vi "Write Base Actor DVR.vi"(10 "Base Actor DVR":refnum<data-value>, 11 "TEMPLATE Actor in":refnum<class "TEMPLATE Actor.lvclass">) -> (3 "TEMPLATE Actor out":refnum<class "TEMPLATE Actor.lvclass">)   [LabVIEW 2020, in "_Template.lvlib" / "Templates.lvlib" / "TEMPLATE jettl Actor.lvlib" / "TEMPLATE Actor.lvlib" / "TEMPLATE Actor.lvclass"]
uses:
  TEMPLATE Actor.lvclass
  TEMPLATE Actor.lvclass/TEMPLATE Actor.ctl
  jettl/jettl/Unified Actor Lifetime.ctl
  jettl/jettl/jettl.lvlib
  jettl/jettl/Base Actor.ctl
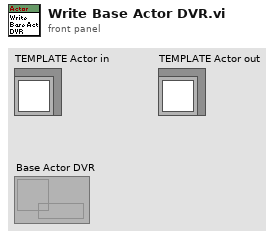
[diagram p1: front panel]
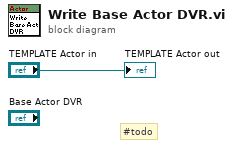
[diagram p0: block diagram]
diagram:
  # "#todo"
  "TEMPLATE Actor out" <- "TEMPLATE Actor in"
